vi "RunSimulationBattery-Detector.vi"() -> ()   [LabVIEW 2019]
uses:
  File Exists - Scalar__ogtk.vi
  <vilib>/Utility/file.llb/Read Delimited Spreadsheet (string).vi
  <vilib>/Utility/file.llb/Write Delimited Spreadsheet (string).vi
  <vilib>/Analysis/NI_AALBase.lvlib
panel:
  out "Time to End":cluster{"Time To End":dbl, "unit":string}={"Time To End"=7.502362424242424, "unit"="hr"} {"Time To End" format="%#_4g"}
  in  "A":dbl[](array[numeric])=[0.0, 0.01, 0.01778279410038923, 0.0316227766016838, 0.056234132519034905, 0.1, 0.1778279410038923, 0.31622776601683794, 0.5623413251903492, 1.0, 1.7782794100389228, 3.1622776601683795, 5.623413251903491, 10.0]
  in  "WD":dbl[](array[numeric])=[1.0, 1.5, 2.0, 2.5, 3.0]
  in  "NA":dbl[](array[numeric])=[0.8, 0.85, 0.9, 0.95, 1.0, 1.05, 1.1, 1.15, 1.2000000000000002]
  out "error out":errorcluster
  in  "Target File":path=path "D:/Ian_s Dropbox/Dropbox/PostDoc/Programs/Data/2020-01-15 BigSlab2 Results v01"
  out "Header":string[](array[string])=["Format Version", "Geometry", "Radius (mm)", "Starting Depth (mm)", "G", "Scattering Coefficient", "Absorption Coefficient", "Simulation Grain (mm)", "START Position X", "START Position Y", "START Position Z", "N Photons", "NA", "WD", "LowScatter - N", "LowScatter - Mean Dist", "LowScatter - SD Dist", "LowScatter - I: A = 0.000000", "LowScatter - I: A = 0.010000", "LowScatter - I: A = 0.017783", "LowScatter - I: A = 0.031623", "LowScatter - I: A = 0.056234", "LowScatter - I: A = 0.100000", "LowScatter - I: A = 0.177828", "LowScatter - I: A = 0.316228", "LowScatter - I: A = 0.562341", "LowScatter - I: A = 1.000000", "LowScatter - I: A = 1.778279", "LowScatter - I: A = 3.162278", "LowScatter - I: A = 5.623413", "LowScatter - I: A = 10.000000", "LowScatter - Ave(I): A = 0.000000", "LowScatter - Ave(I): A = 0.010000", "LowScatter - Ave(I): A = 0.017783", "LowScatter - Ave(I): A = 0.031623", "LowScatter - Ave(I): A = 0.056234", "LowScatter - Ave(I): A = 0.100000", "LowScatter - Ave(I): A = 0.177828", "LowScatter - Ave(I): A = 0.316228", "LowScatter - Ave(I): A = 0.562341", "LowScatter - Ave(I): A = 1.000000", "LowScatter - Ave(I): A = 1.778279", "LowScatter - Ave(I): A = 3.162278", "LowScatter - Ave(I): A = 5.623413", "LowScatter - Ave(I): A = 10.000000", "LowScatter - SD(I): A = 0.000000", "LowScatter - SD(I): A = 0.010000", "LowScatter - SD(I): A = 0.017783", "LowScatter - SD(I): A = 0.031623", "LowScatter - SD(I): A = 0.056234", "LowScatter - SD(I): A = 0.100000", "LowScatter - SD(I): A = 0.177828", "LowScatter - SD(I): A = 0.316228", "LowScatter - SD(I): A = 0.562341", "LowScatter - SD(I): A = 1.000000", "LowScatter - SD(I): A = 1.778279", "LowScatter - SD(I): A = 3.162278", "LowScatter - SD(I): A = 5.623413", "LowScatter - SD(I): A = 10.000000"]
  out "transposed array":string[][](array[string])=[["Format Version", "Geometry", "Radius (mm)", "Starting Depth (mm)", "G", "Scattering Coefficient", "Absorption Coefficient", "Simulation Grain (mm)", "START Position X", "START Position Y", "START Position Z"], ["2.0", "SLAB", "5.000000E+0", "1.000000E-9", "9.200000E-1", "0.000000E+0", "1.000000E+0", "1.000000E-4", "0.000000E+0", "0.000000E+0", "5.000000E+0"]]
  out "file names":string[](array[string])=["BigSlab2--SLAB--R5--D0--G0.92--S0--A1--grain0.0001.txt", "BigSlab2--SLAB--R5--D0--G0.92--S0.1--A1--grain0.0001.txt", "BigSlab2--SLAB--R5--D0--G0.92--S0.177828--A1--grain0.0001.txt", "BigSlab2--SLAB--R5--D0--G0.92--S0.316228--A1--grain0.0001.txt", "BigSlab2--SLAB--R5--D0--G0.92--S0.562341--A1--grain0.0001.txt", "BigSlab2--SLAB--R5--D0--G0.92--S1--A1--grain0.0001.txt", "BigSlab2--SLAB--R5--D0--G0.92--S1.778279--A1--grain0.0001.txt", "BigSlab2--SLAB--R5--D0--G0.92--S10--A1--grain0.0001.txt", "BigSlab2--SLAB--R5--D0--G0.92--S3.162278--A1--grain0.0001.txt", "BigSlab2--SLAB--R5--D0--G0.92--S5.623413--A1--grain0.0001.txt", "BigSlab2--SLAB--R5--D0.1--G0.92--S0--A1--grain0.0001.txt", "BigSlab2--SLAB--R5--D0.1--G0.92--S0.1--A1--grain0.0001.txt", "BigSlab2--SLAB--R5--D0.1--G0.92--S0.177828--A1--grain0.0001.txt", "BigSlab2--SLAB--R5--D0.1--G0.92--S0.316228--A1--grain0.0001.txt", "BigSlab2--SLAB--R5--D0.1--G0.92--S0.562341--A1--grain0.0001.txt", "BigSlab2--SLAB--R5--D0.1--G0.92--S1--A1--grain0.0001.txt", "BigSlab2--SLAB--R5--D0.1--G0.92--S1.778279--A1--grain0.0001.txt", "BigSlab2--SLAB--R5--D0.1--G0.92--S10--A1--grain0.0001.txt", "BigSlab2--SLAB--R5--D0.1--G0.92--S3.162278--A1--grain0.0001.txt", "BigSlab2--SLAB--R5--D0.1--G0.92--S5.623413--A1--grain0.0001.txt", "BigSlab2--SLAB--R5--D0.2--G0.92--S0--A1--grain0.0001.txt", "BigSlab2--SLAB--R5--D0.2--G0.92--S0.1--A1--grain0.0001.txt", "BigSlab2--SLAB--R5--D0.2--G0.92--S0.177828--A1--grain0.0001.txt", "BigSlab2--SLAB--R5--D0.2--G0.92--S0.316228--A1--grain0.0001.txt", "BigSlab2--SLAB--R5--D0.2--G0.92--S0.562341--A1--grain0.0001.txt", "BigSlab2--SLAB--R5--D0.2--G0.92--S1--A1--grain0.0001.txt", "BigSlab2--SLAB--R5--D0.2--G0.92--S1.778279--A1--grain0.0001.txt", "BigSlab2--SLAB--R5--D0.2--G0.92--S10--A1--grain0.0001.txt", "BigSlab2--SLAB--R5--D0.2--G0.92--S3.162278--A1--grain0.0001.txt", "BigSlab2--SLAB--R5--D0.2--G0.92--S5.623413--A1--grain0.0001.txt", "BigSlab2--SLAB--R5--D0.3--G0.92--S0--A1--grain0.0001.txt", "BigSlab2--SLAB--R5--D0.3--G0.92--S0.1--A1--grain0.0001.txt", "BigSlab2--SLAB--R5--D0.3--G0.92--S0.177828--A1--grain0.0001.txt", "BigSlab2--SLAB--R5--D0.3--G0.92--S0.316228--A1--grain0.0001.txt", "BigSlab2--SLAB--R5--D0.3--G0.92--S0.562341--A1--grain0.0001.txt", "BigSlab2--SLAB--R5--D0.3--G0.92--S1--A1--grain0.0001.txt", "BigSlab2--SLAB--R5--D0.3--G0.92--S1.778279--A1--grain0.0001.txt", "BigSlab2--SLAB--R5--D0.3--G0.92--S10--A1--grain0.0001.txt", "BigSlab2--SLAB--R5--D0.3--G0.92--S3.162278--A1--grain0.0001.txt", "BigSlab2--SLAB--R5--D0.3--G0.92--S5.623413--A1--grain0.0001.txt", "BigSlab2--SLAB--R5--D0.4--G0.92--S0--A1--grain0.0001.txt", "BigSlab2--SLAB--R5--D0.4--G0.92--S0.1--A1--grain0.0001.txt", "BigSlab2--SLAB--R5--D0.4--G0.92--S0.177828--A1--grain0.0001.txt", "BigSlab2--SLAB--R5--D0.4--G0.92--S0.316228--A1--grain0.0001.txt", "BigSlab2--SLAB--R5--D0.4--G0.92--S0.562341--A1--grain0.0001.txt", "BigSlab2--SLAB--R5--D0.4--G0.92--S1--A1--grain0.0001.txt", "BigSlab2--SLAB--R5--D0.4--G0.92--S1.778279--A1--grain0.0001.txt", "BigSlab2--SLAB--R5--D0.4--G0.92--S10--A1--grain0.0001.txt", "BigSlab2--SLAB--R5--D0.4--G0.92--S3.162278--A1--grain0.0001.txt", "BigSlab2--SLAB--R5--D0.4--G0.92--S5.623413--A1--grain0.0001.txt", "BigSlab2--SLAB--R5--D0.5--G0.92--S0--A1--grain0.0001.txt", "BigSlab2--SLAB--R5--D0.5--G0.92--S0.1--A1--grain0.0001.txt", "BigSlab2--SLAB--R5--D0.5--G0.92--S0.177828--A1--grain0.0001.txt", "BigSlab2--SLAB--R5--D0.5--G0.92--S0.316228--A1--grain0.0001.txt", "BigSlab2--SLAB--R5--D0.5--G0.92--S0.562341--A1--grain0.0001.txt", "BigSlab2--SLAB--R5--D0.5--G0.92--S1--A1--grain0.0001.txt", "BigSlab2--SLAB--R5--D0.5--G0.92--S1.778279--A1--grain0.0001.txt", "BigSlab2--SLAB--R5--D0.5--G0.92--S10--A1--grain0.0001.txt", "BigSlab2--SLAB--R5--D0.5--G0.92--S3.162278--A1--grain0.0001.txt", "BigSlab2--SLAB--R5--D0.5--G0.92--S5.623413--A1--grain0.0001.txt", "BigSlab2--SLAB--R5--D0.6--G0.92--S0--A1--grain0.0001.txt", "BigSlab2--SLAB--R5--D0.6--G0.92--S0.1--A1--grain0.0001.txt", "BigSlab2--SLAB--R5--D0.6--G0.92--S0.177828--A1--grain0.0001.txt", "BigSlab2--SLAB--R5--D0.6--G0.92--S0.316228--A1--grain0.0001.txt", "BigSlab2--SLAB--R5--D0.6--G0.92--S0.562341--A1--grain0.0001.txt", "BigSlab2--SLAB--R5--D0.6--G0.92--S1--A1--grain0.0001.txt", "BigSlab2--SLAB--R5--D0.6--G0.92--S1.778279--A1--grain0.0001.txt", "BigSlab2--SLAB--R5--D0.6--G0.92--S10--A1--grain0.0001.txt", "BigSlab2--SLAB--R5--D0.6--G0.92--S3.162278--A1--grain0.0001.txt", "BigSlab2--SLAB--R5--D0.6--G0.92--S5.623413--A1--grain0.0001.txt", "BigSlab2--SLAB--R5--D0.7--G0.92--S0--A1--grain0.0001.txt", "BigSlab2--SLAB--R5--D0.7--G0.92--S0.1--A1--grain0.0001.txt", "BigSlab2--SLAB--R5--D0.7--G0.92--S0.177828--A1--grain0.0001.txt", "BigSlab2--SLAB--R5--D0.7--G0.92--S0.316228--A1--grain0.0001.txt", "BigSlab2--SLAB--R5--D0.7--G0.92--S0.562341--A1--grain0.0001.txt", "BigSlab2--SLAB--R5--D0.7--G0.92--S1--A1--grain0.0001.txt", "BigSlab2--SLAB--R5--D0.7--G0.92--S1.778279--A1--grain0.0001.txt", "BigSlab2--SLAB--R5--D0.7--G0.92--S10--A1--grain0.0001.txt", "BigSlab2--SLAB--R5--D0.7--G0.92--S3.162278--A1--grain0.0001.txt", "BigSlab2--SLAB--R5--D0.7--G0.92--S5.623413--A1--grain0.0001.txt", "BigSlab2--SLAB--R5--D0.8--G0.92--S0--A1--grain0.0001.txt", "BigSlab2--SLAB--R5--D0.8--G0.92--S0.1--A1--grain0.0001.txt", "BigSlab2--SLAB--R5--D0.8--G0.92--S0.177828--A1--grain0.0001.txt", "BigSlab2--SLAB--R5--D0.8--G0.92--S0.316228--A1--grain0.0001.txt", "BigSlab2--SLAB--R5--D0.8--G0.92--S0.562341--A1--grain0.0001.txt", "BigSlab2--SLAB--R5--D0.8--G0.92--S1--A1--grain0.0001.txt", "BigSlab2--SLAB--R5--D0.8--G0.92--S1.778279--A1--grain0.0001.txt", "BigSlab2--SLAB--R5--D0.8--G0.92--S10--A1--grain0.0001.txt", "BigSlab2--SLAB--R5--D0.8--G0.92--S3.162278--A1--grain0.0001.txt", "BigSlab2--SLAB--R5--D0.8--G0.92--S5.623413--A1--grain0.0001.txt", "BigSlab2--SLAB--R5--D0.9--G0.92--S0--A1--grain0.0001.txt", "BigSlab2--SLAB--R5--D0.9--G0.92--S0.1--A1--grain0.0001.txt", "BigSlab2--SLAB--R5--D0.9--G0.92--S0.177828--A1--grain0.0001.txt", "BigSlab2--SLAB--R5--D0.9--G0.92--S0.316228--A1--grain0.0001.txt", "BigSlab2--SLAB--R5--D0.9--G0.92--S0.562341--A1--grain0.0001.txt", "BigSlab2--SLAB--R5--D0.9--G0.92--S1--A1--grain0.0001.txt", "BigSlab2--SLAB--R5--D0.9--G0.92--S1.778279--A1--grain0.0001.txt", "BigSlab2--SLAB--R5--D0.9--G0.92--S10--A1--grain0.0001.txt", "BigSlab2--SLAB--R5--D0.9--G0.92--S3.162278--A1--grain0.0001.txt", "BigSlab2--SLAB--R5--D0.9--G0.92--S5.623413--A1--grain0.0001.txt", "BigSlab2--SLAB--R5--D1--G0.92--S0--A1--grain0.0001.txt", "BigSlab2--SLAB--R5--D1--G0.92--S0.1--A1--grain0.0001.txt", "BigSlab2--SLAB--R5--D1--G0.92--S0.177828--A1--grain0.0001.txt", "BigSlab2--SLAB--R5--D1--G0.92--S0.316228--A1--grain0.0001.txt", "BigSlab2--SLAB--R5--D1--G0.92--S0.562341--A1--grain0.0001.txt", "BigSlab2--SLAB--R5--D1--G0.92--S1--A1--grain0.0001.txt", "BigSlab2--SLAB--R5--D1--G0.92--S1.778279--A1--grain0.0001.txt", "BigSlab2--SLAB--R5--D1--G0.92--S10--A1--grain0.0001.txt", "BigSlab2--SLAB--R5--D1--G0.92--S3.162278--A1--grain0.0001.txt", "BigSlab2--SLAB--R5--D1--G0.92--S5.623413--A1--grain0.0001.txt", "BigSlab2--SLAB--R5--D1.1--G0.92--S0--A1--grain0.0001.txt", "BigSlab2--SLAB--R5--D1.1--G0.92--S0.1--A1--grain0.0001.txt", "BigSlab2--SLAB--R5--D1.1--G0.92--S0.177828--A1--grain0.0001.txt", "BigSlab2--SLAB--R5--D1.1--G0.92--S0.316228--A1--grain0.0001.txt", "BigSlab2--SLAB--R5--D1.1--G0.92--S0.562341--A1--grain0.0001.txt", "BigSlab2--SLAB--R5--D1.1--G0.92--S1--A1--grain0.0001.txt", "BigSlab2--SLAB--R5--D1.1--G0.92--S1.778279--A1--grain0.0001.txt", "BigSlab2--SLAB--R5--D1.1--G0.92--S10--A1--grain0.0001.txt", "BigSlab2--SLAB--R5--D1.1--G0.92--S3.162278--A1--grain0.0001.txt", "BigSlab2--SLAB--R5--D1.1--G0.92--S5.623413--A1--grain0.0001.txt", "BigSlab2--SLAB--R5--D1.2--G0.92--S0--A1--grain0.0001.txt", "BigSlab2--SLAB--R5--D1.2--G0.92--S0.1--A1--grain0.0001.txt", "BigSlab2--SLAB--R5--D1.2--G0.92--S0.177828--A1--grain0.0001.txt", "BigSlab2--SLAB--R5--D1.2--G0.92--S0.316228--A1--grain0.0001.txt", "BigSlab2--SLAB--R5--D1.2--G0.92--S0.562341--A1--grain0.0001.txt", "BigSlab2--SLAB--R5--D1.2--G0.92--S1--A1--grain0.0001.txt", "BigSlab2--SLAB--R5--D1.2--G0.92--S1.778279--A1--grain0.0001.txt", "BigSlab2--SLAB--R5--D1.2--G0.92--S10--A1--grain0.0001.txt", "BigSlab2--SLAB--R5--D1.2--G0.92--S3.162278--A1--grain0.0001.txt", "BigSlab2--SLAB--R5--D1.2--G0.92--S5.623413--A1--grain0.0001.txt", "BigSlab2--SLAB--R5--D1.3--G0.92--S0--A1--grain0.0001.txt", "BigSlab2--SLAB--R5--D1.3--G0.92--S0.1--A1--grain0.0001.txt", "BigSlab2--SLAB--R5--D1.3--G0.92--S0.177828--A1--grain0.0001.txt", "BigSlab2--SLAB--R5--D1.3--G0.92--S0.316228--A1--grain0.0001.txt", "BigSlab2--SLAB--R5--D1.3--G0.92--S0.562341--A1--grain0.0001.txt", "BigSlab2--SLAB--R5--D1.3--G0.92--S1--A1--grain0.0001.txt", "BigSlab2--SLAB--R5--D1.3--G0.92--S1.778279--A1--grain0.0001.txt", "BigSlab2--SLAB--R5--D1.3--G0.92--S10--A1--grain0.0001.txt", "BigSlab2--SLAB--R5--D1.3--G0.92--S3.162278--A1--grain0.0001.txt", "BigSlab2--SLAB--R5--D1.3--G0.92--S5.623413--A1--grain0.0001.txt", "BigSlab2--SLAB--R5--D1.4--G0.92--S0--A1--grain0.0001.txt", "BigSlab2--SLAB--R5--D1.4--G0.92--S0.1--A1--grain0.0001.txt", "BigSlab2--SLAB--R5--D1.4--G0.92--S0.177828--A1--grain0.0001.txt", "BigSlab2--SLAB--R5--D1.4--G0.92--S0.316228--A1--grain0.0001.txt", "BigSlab2--SLAB--R5--D1.4--G0.92--S0.562341--A1--grain0.0001.txt", "BigSlab2--SLAB--R5--D1.4--G0.92--S1--A1--grain0.0001.txt", "BigSlab2--SLAB--R5--D1.4--G0.92--S1.778279--A1--grain0.0001.txt", "BigSlab2--SLAB--R5--D1.4--G0.92--S10--A1--grain0.0001.txt", "BigSlab2--SLAB--R5--D1.4--G0.92--S3.162278--A1--grain0.0001.txt", "BigSlab2--SLAB--R5--D1.4--G0.92--S5.623413--A1--grain0.0001.txt", "BigSlab2--SLAB--R5--D1.5--G0.92--S0--A1--grain0.0001.txt", "BigSlab2--SLAB--R5--D1.5--G0.92--S0.1--A1--grain0.0001.txt", "BigSlab2--SLAB--R5--D1.5--G0.92--S0.177828--A1--grain0.0001.txt", "BigSlab2--SLAB--R5--D1.5--G0.92--S0.316228--A1--grain0.0001.txt", "BigSlab2--SLAB--R5--D1.5--G0.92--S0.562341--A1--grain0.0001.txt", "BigSlab2--SLAB--R5--D1.5--G0.92--S1--A1--grain0.0001.txt", "BigSlab2--SLAB--R5--D1.5--G0.92--S1.778279--A1--grain0.0001.txt", "BigSlab2--SLAB--R5--D1.5--G0.92--S10--A1--grain0.0001.txt", "BigSlab2--SLAB--R5--D1.5--G0.92--S3.162278--A1--grain0.0001.txt", "BigSlab2--SLAB--R5--D1.5--G0.92--S5.623413--A1--grain0.0001.txt", "BigSlab2--SLAB--R5--D1.6--G0.92--S0--A1--grain0.0001.txt", "BigSlab2--SLAB--R5--D1.6--G0.92--S0.1--A1--grain0.0001.txt", "BigSlab2--SLAB--R5--D1.6--G0.92--S0.177828--A1--grain0.0001.txt", "BigSlab2--SLAB--R5--D1.6--G0.92--S0.316228--A1--grain0.0001.txt", "BigSlab2--SLAB--R5--D1.6--G0.92--S0.562341--A1--grain0.0001.txt", "BigSlab2--SLAB--R5--D1.6--G0.92--S1--A1--grain0.0001.txt", "BigSlab2--SLAB--R5--D1.6--G0.92--S1.778279--A1--grain0.0001.txt", "BigSlab2--SLAB--R5--D1.6--G0.92--S10--A1--grain0.0001.txt", "BigSlab2--SLAB--R5--D1.6--G0.92--S3.162278--A1--grain0.0001.txt", "BigSlab2--SLAB--R5--D1.6--G0.92--S5.623413--A1--grain0.0001.txt", "BigSlab2--SLAB--R5--D1.7--G0.92--S0--A1--grain0.0001.txt", "BigSlab2--SLAB--R5--D1.7--G0.92--S0.1--A1--grain0.0001.txt", "BigSlab2--SLAB--R5--D1.7--G0.92--S0.177828--A1--grain0.0001.txt", "BigSlab2--SLAB--R5--D1.7--G0.92--S0.316228--A1--grain0.0001.txt", "BigSlab2--SLAB--R5--D1.7--G0.92--S0.562341--A1--grain0.0001.txt", "BigSlab2--SLAB--R5--D1.7--G0.92--S1--A1--grain0.0001.txt", "BigSlab2--SLAB--R5--D1.7--G0.92--S1.778279--A1--grain0.0001.txt", "BigSlab2--SLAB--R5--D1.7--G0.92--S10--A1--grain0.0001.txt", "BigSlab2--SLAB--R5--D1.7--G0.92--S3.162278--A1--grain0.0001.txt", "BigSlab2--SLAB--R5--D1.7--G0.92--S5.623413--A1--grain0.0001.txt", "BigSlab2--SLAB--R5--D1.8--G0.92--S0--A1--grain0.0001.txt", "BigSlab2--SLAB--R5--D1.8--G0.92--S0.1--A1--grain0.0001.txt", "BigSlab2--SLAB--R5--D1.8--G0.92--S0.177828--A1--grain0.0001.txt", "BigSlab2--SLAB--R5--D1.8--G0.92--S0.316228--A1--grain0.0001.txt", "BigSlab2--SLAB--R5--D1.8--G0.92--S0.562341--A1--grain0.0001.txt", "BigSlab2--SLAB--R5--D1.8--G0.92--S1--A1--grain0.0001.txt", "BigSlab2--SLAB--R5--D1.8--G0.92--S1.778279--A1--grain0.0001.txt", "BigSlab2--SLAB--R5--D1.8--G0.92--S10--A1--grain0.0001.txt", "BigSlab2--SLAB--R5--D1.8--G0.92--S3.162278--A1--grain0.0001.txt", "BigSlab2--SLAB--R5--D1.8--G0.92--S5.623413--A1--grain0.0001.txt", "BigSlab2--SLAB--R5--D1.9--G0.92--S0--A1--grain0.0001.txt", "BigSlab2--SLAB--R5--D1.9--G0.92--S0.1--A1--grain0.0001.txt", "BigSlab2--SLAB--R5--D1.9--G0.92--S0.177828--A1--grain0.0001.txt", "BigSlab2--SLAB--R5--D1.9--G0.92--S0.316228--A1--grain0.0001.txt", "BigSlab2--SLAB--R5--D1.9--G0.92--S0.562341--A1--grain0.0001.txt", "BigSlab2--SLAB--R5--D1.9--G0.92--S1--A1--grain0.0001.txt", "BigSlab2--SLAB--R5--D1.9--G0.92--S1.778279--A1--grain0.0001.txt", "BigSlab2--SLAB--R5--D1.9--G0.92--S10--A1--grain0.0001.txt", "BigSlab2--SLAB--R5--D1.9--G0.92--S3.162278--A1--grain0.0001.txt", "BigSlab2--SLAB--R5--D1.9--G0.92--S5.623413--A1--grain0.0001.txt", "BigSlab2--SLAB--R5--D2--G0.92--S0--A1--grain0.0001.txt", "BigSlab2--SLAB--R5--D2--G0.92--S0.1--A1--grain0.0001.txt", "BigSlab2--SLAB--R5--D2--G0.92--S0.177828--A1--grain0.0001.txt", "BigSlab2--SLAB--R5--D2--G0.92--S0.316228--A1--grain0.0001.txt", "BigSlab2--SLAB--R5--D2--G0.92--S0.562341--A1--grain0.0001.txt", "BigSlab2--SLAB--R5--D2--G0.92--S1--A1--grain0.0001.txt", "BigSlab2--SLAB--R5--D2--G0.92--S1.778279--A1--grain0.0001.txt", "BigSlab2--SLAB--R5--D2--G0.92--S10--A1--grain0.0001.txt", "BigSlab2--SLAB--R5--D2--G0.92--S3.162278--A1--grain0.0001.txt", "BigSlab2--SLAB--R5--D2--G0.92--S5.623413--A1--grain0.0001.txt", "BigSlab2--SLAB--R5--D2.5--G0.92--S0--A1--grain0.0001.txt", "BigSlab2--SLAB--R5--D2.5--G0.92--S0.1--A1--grain0.0001.txt", "BigSlab2--SLAB--R5--D2.5--G0.92--S0.177828--A1--grain0.0001.txt", "BigSlab2--SLAB--R5--D2.5--G0.92--S0.316228--A1--grain0.0001.txt", "BigSlab2--SLAB--R5--D2.5--G0.92--S0.562341--A1--grain0.0001.txt", "BigSlab2--SLAB--R5--D2.5--G0.92--S1--A1--grain0.0001.txt", "BigSlab2--SLAB--R5--D2.5--G0.92--S1.778279--A1--grain0.0001.txt", "BigSlab2--SLAB--R5--D2.5--G0.92--S10--A1--grain0.0001.txt", "BigSlab2--SLAB--R5--D2.5--G0.92--S3.162278--A1--grain0.0001.txt", "BigSlab2--SLAB--R5--D2.5--G0.92--S5.623413--A1--grain0.0001.txt", "BigSlab2--SLAB--R5--D3--G0.92--S0--A1--grain0.0001.txt", "BigSlab2--SLAB--R5--D3--G0.92--S0.1--A1--grain0.0001.txt", "BigSlab2--SLAB--R5--D3--G0.92--S0.177828--A1--grain0.0001.txt", "BigSlab2--SLAB--R5--D3--G0.92--S0.316228--A1--grain0.0001.txt", "BigSlab2--SLAB--R5--D3--G0.92--S0.562341--A1--grain0.0001.txt", "BigSlab2--SLAB--R5--D3--G0.92--S1--A1--grain0.0001.txt", "BigSlab2--SLAB--R5--D3--G0.92--S1.778279--A1--grain0.0001.txt", "BigSlab2--SLAB--R5--D3--G0.92--S10--A1--grain0.0001.txt", "BigSlab2--SLAB--R5--D3--G0.92--S3.162278--A1--grain0.0001.txt", "BigSlab2--SLAB--R5--D3--G0.92--S5.623413--A1--grain0.0001.txt", "BigSlab2--SLAB--R5--D3.5--G0.92--S0--A1--grain0.0001.txt", "BigSlab2--SLAB--R5--D3.5--G0.92--S0.1--A1--grain0.0001.txt", "BigSlab2--SLAB--R5--D3.5--G0.92--S0.177828--A1--grain0.0001.txt", "BigSlab2--SLAB--R5--D3.5--G0.92--S0.316228--A1--grain0.0001.txt", "BigSlab2--SLAB--R5--D3.5--G0.92--S0.562341--A1--grain0.0001.txt", "BigSlab2--SLAB--R5--D3.5--G0.92--S1--A1--grain0.0001.txt", "BigSlab2--SLAB--R5--D3.5--G0.92--S1.778279--A1--grain0.0001.txt", "BigSlab2--SLAB--R5--D3.5--G0.92--S10--A1--grain0.0001.txt", "BigSlab2--SLAB--R5--D3.5--G0.92--S3.162278--A1--grain0.0001.txt", "BigSlab2--SLAB--R5--D3.5--G0.92--S5.623413--A1--grain0.0001.txt", "BigSlab2--SLAB--R5--D4--G0.92--S0--A1--grain0.0001.txt", "BigSlab2--SLAB--R5--D4--G0.92--S0.1--A1--grain0.0001.txt", "BigSlab2--SLAB--R5--D4--G0.92--S0.177828--A1--grain0.0001.txt", "BigSlab2--SLAB--R5--D4--G0.92--S0.316228--A1--grain0.0001.txt", "BigSlab2--SLAB--R5--D4--G0.92--S0.562341--A1--grain0.0001.txt", "BigSlab2--SLAB--R5--D4--G0.92--S1--A1--grain0.0001.txt", "BigSlab2--SLAB--R5--D4--G0.92--S1.778279--A1--grain0.0001.txt", "BigSlab2--SLAB--R5--D4--G0.92--S10--A1--grain0.0001.txt", "BigSlab2--SLAB--R5--D4--G0.92--S3.162278--A1--grain0.0001.txt", "BigSlab2--SLAB--R5--D4--G0.92--S5.623413--A1--grain0.0001.txt", "BigSlab2--SLAB--R5--D4.5--G0.92--S0--A1--grain0.0001.txt", "BigSlab2--SLAB--R5--D4.5--G0.92--S0.1--A1--grain0.0001.txt", "BigSlab2--SLAB--R5--D4.5--G0.92--S0.177828--A1--grain0.0001.txt", "BigSlab2--SLAB--R5--D4.5--G0.92--S0.316228--A1--grain0.0001.txt", "BigSlab2--SLAB--R5--D4.5--G0.92--S0.562341--A1--grain0.0001.txt", "BigSlab2--SLAB--R5--D4.5--G0.92--S1--A1--grain0.0001.txt", "BigSlab2--SLAB--R5--D4.5--G0.92--S1.778279--A1--grain0.0001.txt", "BigSlab2--SLAB--R5--D4.5--G0.92--S10--A1--grain0.0001.txt", "BigSlab2--SLAB--R5--D4.5--G0.92--S3.162278--A1--grain0.0001.txt", "BigSlab2--SLAB--R5--D4.5--G0.92--S5.623413--A1--grain0.0001.txt", "BigSlab2--SLAB--R5--D5--G0.92--S0--A1--grain0.0001.txt", "BigSlab2--SLAB--R5--D5--G0.92--S0.1--A1--grain0.0001.txt", "BigSlab2--SLAB--R5--D5--G0.92--S0.177828--A1--grain0.0001.txt", "BigSlab2--SLAB--R5--D5--G0.92--S0.316228--A1--grain0.0001.txt", "BigSlab2--SLAB--R5--D5--G0.92--S0.562341--A1--grain0.0001.txt", "BigSlab2--SLAB--R5--D5--G0.92--S1--A1--grain0.0001.txt", "BigSlab2--SLAB--R5--D5--G0.92--S1.778279--A1--grain0.0001.txt", "BigSlab2--SLAB--R5--D5--G0.92--S10--A1--grain0.0001.txt", "BigSlab2--SLAB--R5--D5--G0.92--S3.162278--A1--grain0.0001.txt", "BigSlab2--SLAB--R5--D5--G0.92--S5.623413--A1--grain0.0001.txt"]
  out "Percent Complete":dbl(slide)=0.0018106995884773663 scale=0.0..1.0
  in  "Folder of Media Simulations":path=path "D:/Ian_s Dropbox/Dropbox/PostDoc/Programs/Data/2020-01-15 BigSlab2"
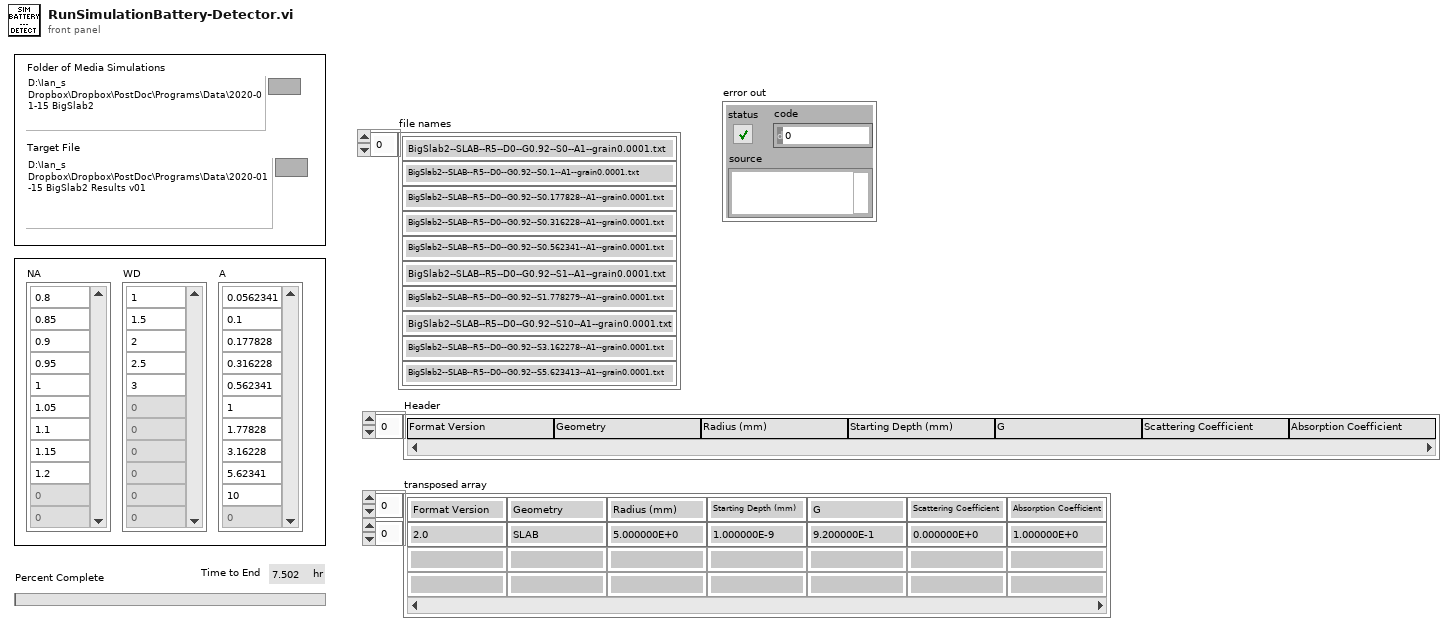
[diagram p1: front panel]
types:
  T1 = enum16{"Delete Empty Rows", "Delete Empty Columns"}
  T2 = typedef "PhotonState--Enum.ctl" = enum16{"Detected - Low Scattering", "Detected - High Scattering", "Undetected"}
  T3 = cluster{"Photon State":T2, "Phi":dbl, "String":dbl}
  T4 = cluster{"Photon State":T2, "Phi":dbl, "String":dbl}[]
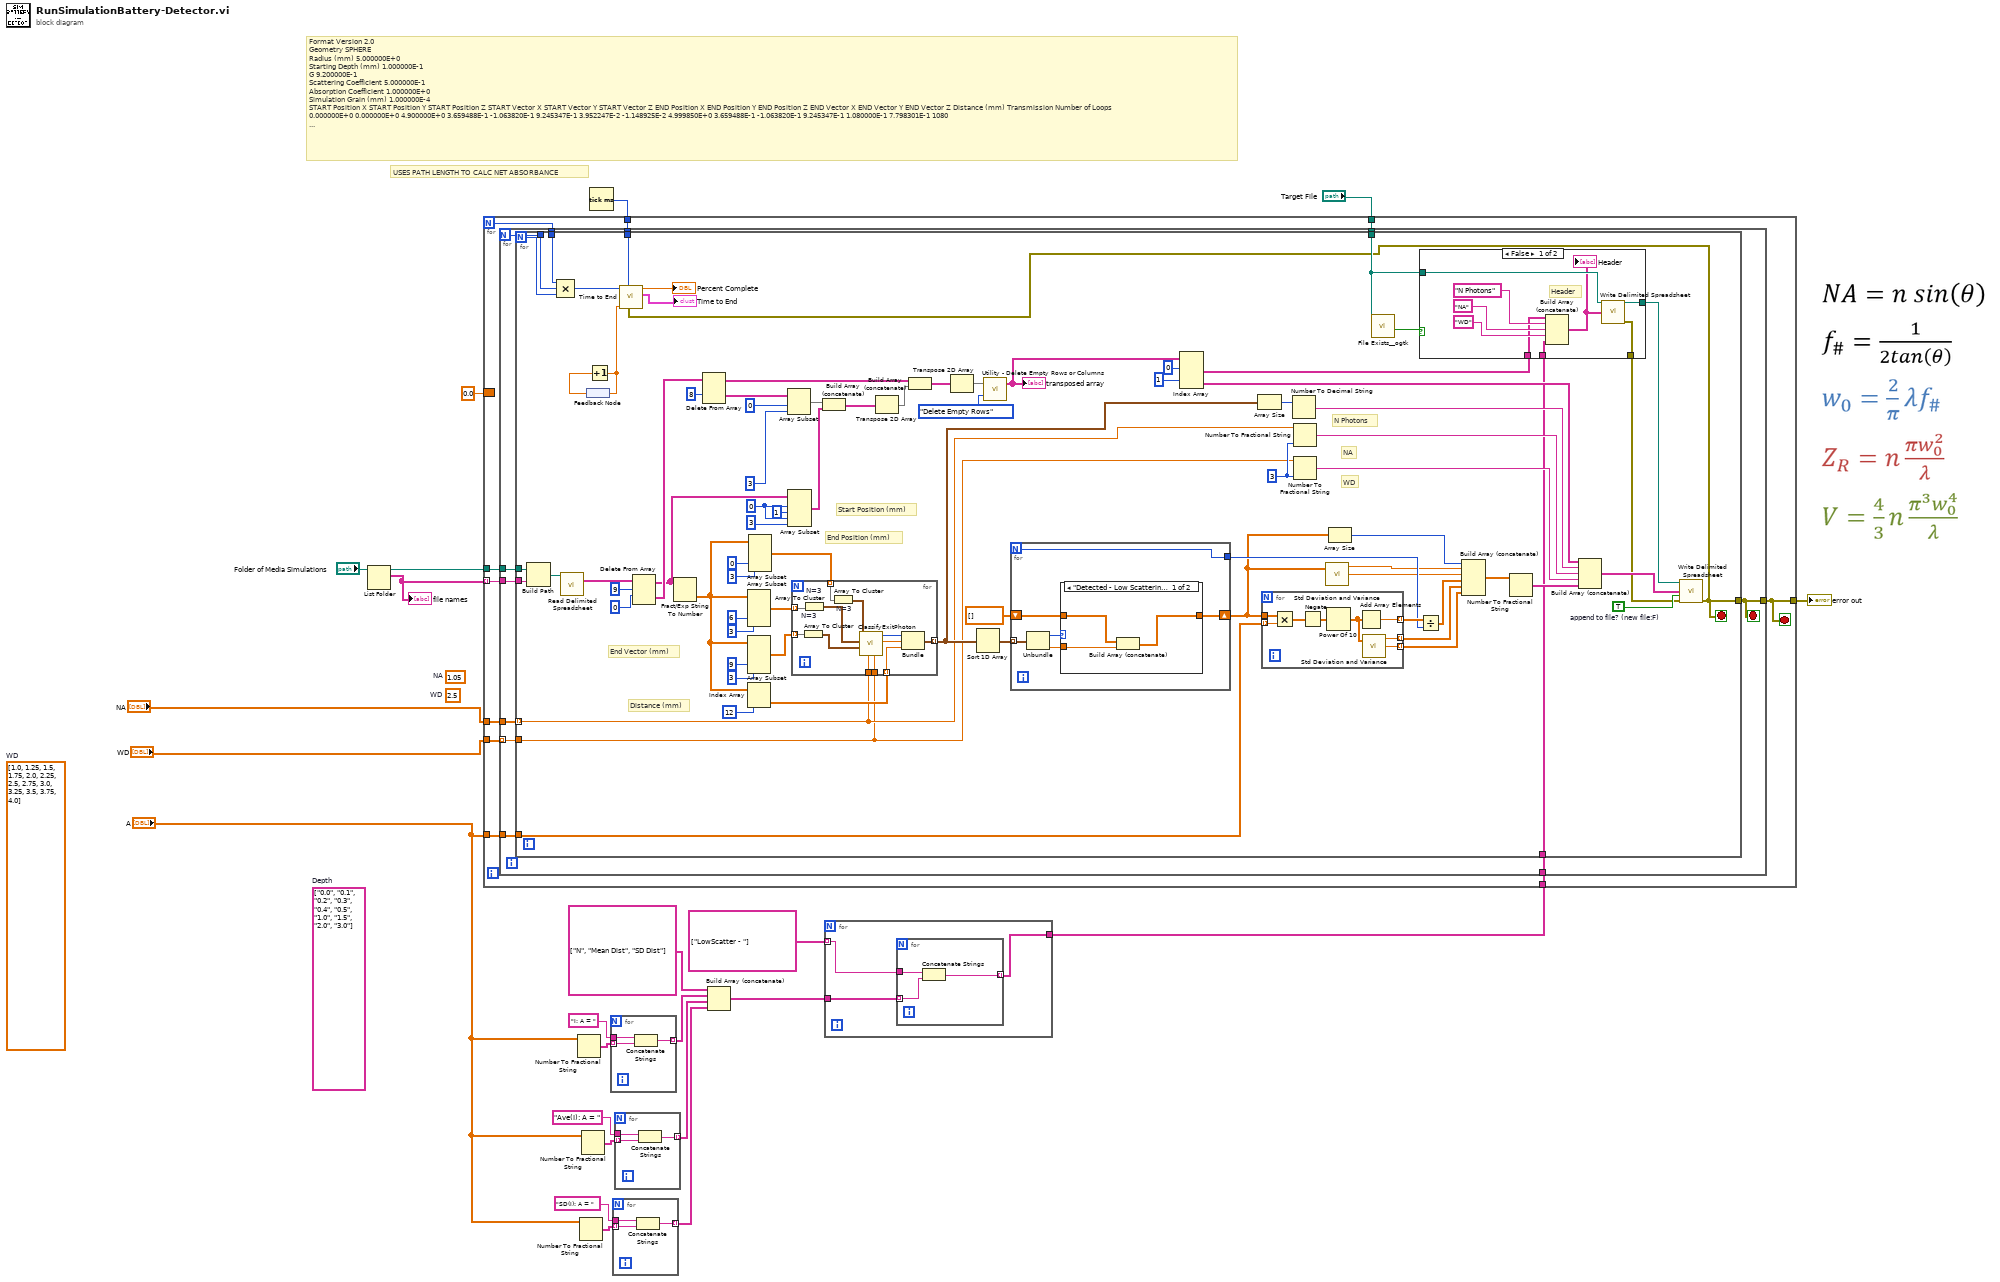
[diagram p0: block diagram]
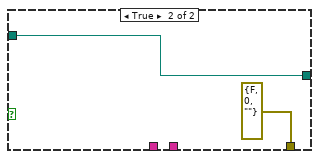
[diagram p2: hidden frame]
diagram:
  (unwired) dbl[] [1.0, 1.25, 1.5, 1.75, 2.0, 2.25, 2.5, 2.75, 3.0, 3.25, 3.5, 3.75, 4.0]  # WD
  (unwired) 2.5  # WD
  (unwired) 1.05  # NA
  (unwired) string[] ["0.0", "0.1", "0.2", "0.3", "0.4", "0.5", "1.0", "1.5", "2.0", "3.0"]  # Depth
  # "Format Version\t2.0\t\t\t\t\t\t\t\t\t\t\t\t\t\nGeometry\tSPHERE\t\t\t\t\t\t\t\t\t\t\t\t\t\nRadius (mm)\t5.000000E+0\t\t\t\t\t\t\t\t\t\t\t\t\t\nStarting Depth (mm)\t1.000000E-1\t\t\t\t\t\t\t\t\t\t\t\t\t\nG\t9.200000E-1\t\t\t\t\t\t\t\t\t\t\t\t\t\nScattering Coefficient\t5.000000E-1\t\t\t\t\t\t\t\t\t\t\t\t\t\nAbsorption Coefficient\t1.000000E+0\t\t\t\t\t\t\t\t\t\t\t\t\t\nSimulation Grain (mm)\t1.000000E-4\t\t\t\t\t\t\t\t\t\t\t\t\t\nSTART Position X\tSTART Position Y\tSTART Position Z\tSTART Vector X\tSTART Vector Y\tSTART Vector Z\tEND Position X\tEND Position Y\tEND Position Z\tEND Vector X\tEND Vector Y\tEND Vector Z\tDistance (mm)\tTransmission\tNumber of Loops\n0.000000E+0\t0.000000E+0\t4.900000E+0\t3.659488E-1\t-1.063820E-1\t9.245347E-1\t3.952247E-2\t-1.148925E-2\t4.999850E+0\t3.659488E-1\t-1.063820E-1\t9.245347E-1\t1.080000E-1\t7.798301E-1\t1080\n..."
  # "USES PATH LENGTH TO CALC NET ABSORBANCE"
  n1 = List Folder(path="Folder of Media Simulations") -> (path out=w21:path, filenames=w22:string[])  [unwired: 3 in, 2 out]
  "file names" <- w22
  n2 = Number To Fractional String(number="A") -> (F-format string=w20:string[])  [unwired: 3 in]
  n3 = Number To Fractional String(number="A") -> (F-format string=w12:string[])  [unwired: 3 in]
  n4 = Number To Fractional String(number="A") -> (F-format string=w13:string[])  [unwired: 3 in]
  n5 = Tick Count (ms)() -> (millisecond timer value=w1:u32)
  n6 = for {
    tunnel: w20 -> [w26] mode=indexing
    tunnel: "I: A = " ("string") -> [w25]
    tunnel: [w24] -> w17 mode=indexing
    n7 = Concatenate Strings(w25, w26) -> (w24:string)
  }
  n8 = for {
    tunnel: w12 -> [w29] mode=indexing
    tunnel: "SD(I): A = " ("string") -> [w28]
    tunnel: [w27] -> w9 mode=indexing
    n9 = Concatenate Strings(w28, w29) -> (w27:string)
  }
  n10 = for {
    tunnel: w13 -> [w32] mode=indexing
    tunnel: "Ave(I): A = " ("string") -> [w31]
    tunnel: [w30] -> w10 mode=indexing
    n11 = Concatenate Strings(w31, w32) -> (w30:string)
  }
  n12 = Build Array (concatenate)(string[] ["N", "Mean Dist", "SD Dist"] ("Array 2"), w17, w10, w9) -> (w15:string[])
  n13 = for {
    tunnel: string[] ["LowScatter - "] ("Array 2") -> [w35] mode=indexing
    tunnel: w15 -> [w34]
    tunnel: [w33] -> w4
    n14 = for {
      tunnel: w35 -> [w38]
      tunnel: w34 -> [w37] mode=indexing
      tunnel: [w36] -> w33 mode=indexing
      n15 = Concatenate Strings(w38, w37) -> (w36:string)
    }
  }
  n16 = for {
    N -> [w43]
    tunnel: w21 -> [w48]
    tunnel: "NA" -> [w47]
    tunnel: "A" -> [w44]
    tunnel: w22 -> [w46] mode=indexing
    tunnel: "WD" -> [w45]
    border: 0.0 -> [_]
    tunnel: [w42] -> w3
    tunnel: "Target File" -> [w41]
    tunnel: w4 -> [w40]
    tunnel: w1 -> [w39]
    stop <- w42 stop-if-true
    n17 = for {
      N -> [w54]
      tunnel: w48 -> [w59]
      tunnel: w47 -> [w58]
      tunnel: w46 -> [w57]
      tunnel: w45 -> [w56] mode=indexing
      tunnel: w44 -> [w55]
      tunnel: w43 -> [w53]
      tunnel: [w52] -> w42
      tunnel: w41 -> [w51]
      tunnel: w40 -> [w50]
      tunnel: w39 -> [w49]
      stop <- w52 stop-if-true
      n18 = for {
        N -> [w86]
        tunnel: w59 -> [w138]
        tunnel: w58 -> [w89] mode=indexing
        tunnel: w57 -> [w126]
        tunnel: w56 -> [w88]
        tunnel: w55 -> [w103]
        tunnel: w54 -> [w85]
        tunnel: w53 -> [w84]
        tunnel: [w64] -> w52
        tunnel: w51 -> [w70]
        tunnel: w50 -> [w72]
        tunnel: w49 -> [w62]
        stop <- w64 stop-if-true
        w83 = TRUE  # append to file? (new file:F)
        w90 = i16 3 ("precision (6)")
        w113 = 0 ("index")
        # "WD"
        # "NA"
        # "N Photons"
        # "End Vector (mm)"
        # "End Position (mm)"
        # "Start Position (mm)"
        # "Distance (mm)"
        n19 = Build Path(base path=w138, name or relative path=w126) -> (appended path=w137:path)
        n20 = Compound Arithmetic op=MULTIPLY(w84, w85, w86) -> (w61:i32)
        n21 = call-poly <vilib>:"Read Delimited Spreadsheet.vi"("file path (dialog if empty)"=w137) -> ("all rows"=w125:string[][])  [unwired: 9 in, 5 out]
        n22 = feedback #1() -> (w87:dbl)
        n23 = Increment(x=w87) -> (x+1=w63:dbl)
        n24 = feedback-in #1(w63) -> ()
        n25 = Delete From Array(array=w125, length=9, index (row)=0) -> (deleted portion=w120:string[][], array with subset deleted=w115:string[][])  [unwired: 1 in]
        n26 = Fract/Exp String To Number(string=w115) -> (number=w122:dbl[][])  [unwired: 3 in, 1 out]
        n27 = Delete From Array(array=w120, index (row)=8) -> (deleted portion=w119:string[], array with subset deleted=w108:string[][])  [unwired: 2 in]
        n28 = Array Subset(array=w122, index (col)=6 ("index"), length (col)=3 ("length")) -> (w131:dbl[][])  [unwired: 2 in]
        n29 = Array Subset(array=w122, index (col)=9 ("index"), length (col)=3 ("length")) -> (w130:dbl[][])  [unwired: 2 in]
        n30 = Index Array(array=w122, index (col)=12 ("disabled index (col)")) -> (element=w116:dbl[])  [unwired: 1 in]
        n31 = Array Subset(array=w122, index (col)=0 ("index"), length (col)=3 ("length")) -> (w127:dbl[][])  [unwired: 2 in]
        n32 = Array Subset(array=w119, index=0, length=3) -> (w111:string[])
        n33 = Array Subset(array=w115, index (row)=w113, length (row)=1 ("length"), index (col)=w113, length (col)=3 ("length")) -> (w110:string[][])
        n34 = for {
          tunnel: w131 -> [w179] mode=indexing
          tunnel: w130 -> [w178] mode=indexing
          tunnel: w116 -> [w175] mode=indexing
          tunnel: [w173] -> w96 mode=indexing
          tunnel: w127 -> [w170] mode=indexing
          tunnel: w89 -> [w172]
          tunnel: w88 -> [w168]
          n35 = Array To Cluster "N=3"(array=w178) -> (cluster=w177:cluster{"[0]":dbl, "[1]":dbl, "[2]":dbl})
          n36 = Array To Cluster "N=3"(array=w179) -> (cluster=w176:cluster{"[0]":dbl, "[1]":dbl, "[2]":dbl})
          n37 = Array To Cluster "N=3"(array=w170) -> (cluster=w169:cluster{"[0]":dbl, "[1]":dbl, "[2]":dbl})
          n38 = call "ClassifyExitPhoton.vi"("WD (4)"=w168, "NA (1)"=w172, "V - Exit"=w177, "R - Exit"=w176, "R - Focal Point"=w169) -> ("Phi"=w174:dbl, "Photon State"=w171:T2)  [unwired: 5 in]
          n39 = Bundle("Photon State"=w171, "Phi"=w174, "String"=w175) -> (w173:T3)  [unwired: 1 in]
        }
        n40 = Build Array (concatenate)(w111, w110) -> (w109:string[][])
        n41 = Transpose 2D Array(2D array=w109) -> (transposed array=w107:string[][])
        n42 = Build Array (concatenate)(w108, w107) -> (w106:string[][])
        n43 = Transpose 2D Array(2D array=w106) -> (transposed array=w104:string[][])
        n44 = Sort 1D Array(array=w96) -> (sorted array=w98:T4)
        n45 = call "Utility - Delete Empty Rows or Columns.vi"("Delete Option"=T1."Delete Empty Rows", "Array In"=w104) -> ("Array Out"=w102:string[][])  [unwired: 1 in]
        "transposed array" <- w102
        n46 = for {
          N -> [w158]
          tunnel: w98 -> [w163] mode=indexing
          shift-right: [w160] -> w67
          shift-left: dbl[] [] -> [w159]
          tunnel: [w158] -> w76
          n47 = Unbundle(w163) -> ("Photon State"=w162:T2, "String"=w161:dbl)  [unwired: 1 out]
          n48 = case shown="\"Detected - Low Scattering\"" w162 {
            tunnel: w161 -> [w166 _]
            tunnel: [w165 w167] -> w160
            tunnel: w159 -> [w164 w167]
            frame "Detected - Low Scattering" {
              n49 = Build Array (concatenate)(w164, w166) -> (w165:dbl[])
            }
            frame Default {
            }
          }
        }
        n50 = Index Array(array=w102, index (row) #1=0 ("index (row)"), index (row) #2=1 ("index (row)")) -> (element #1=w71:string[], element #2=w95:string[])  [unwired: 2 in]
        n51 = Array Size(array=w96) -> (size(s)=w97:i32)
        n52 = for {
          tunnel: w103 -> [w157] mode=indexing
          tunnel: w67 -> [w153]
          tunnel: [w154] -> w99 mode=indexing
          tunnel: [w151] -> w79 mode=indexing
          tunnel: [w150] -> w78 mode=indexing
          n53 = Multiply(x=w153, y=w157) -> (x*y=w156:dbl[])
          n54 = Negate(x=w156) -> (-x=w155:dbl[])
          n55 = Power Of 10(x=w155) -> (10^x=w152:dbl[])
          n56 = Add Array Elements(numeric array=w152) -> (sum=w154:dbl)
          n57 = call <vilib>:"Std Deviation and Variance.vi"("X"=w152) -> ("mean"=w151:dbl, "standard deviation"=w150:dbl)  [unwired: 1 in, 1 out]
        }
        n58 = Number To Decimal String(number=w97) -> (decimal integer string=w94:string)  [unwired: 1 in]
        n59 = Number To Fractional String(number=w89, precision (6)=w90) -> (F-format string=w92:string)  [unwired: 2 in]
        n60 = Number To Fractional String(number=w88, precision (6)=w90) -> (F-format string=w91:string)  [unwired: 2 in]
        n61 = call <vilib>:"Std Deviation and Variance.vi"("X"=w67) -> ("mean"=w75:dbl, "standard deviation"=w74:dbl)  [unwired: 1 in, 1 out]
        n62 = Array Size(array=w67) -> (size(s)=w66:i32)
        n63 = call-poly "File Exists__ogtk.vi"("file path"=w70) -> ("exists"=w73:bool)  [unwired: 6 in, 1 out]
        n64 = case shown="False" w73 {
          tunnel: w72 -> [w144 _]
          tunnel: w71 -> [w143 _]
          tunnel: w70 -> [w142 w149]
          tunnel: [w141 w149] -> w69
          tunnel: [w140 errorcluster {"status"=FALSE, "code"=0, "source"=""} ("error out")] -> w68
          frame False {
            # "Header"
            n65 = Build Array (concatenate)(w143, "N Photons", "NA", "WD", w144) -> (w139:string[])
            "Header" <- w139
            n66 = call-poly <vilib>:"Write Delimited Spreadsheet.vi"("file path (dialog if empty)"=w142, "1D data"=w139) -> ("new file path (Not A Path if cancelled)"=w141:path, "error out"=w140:errorcluster)  [unwired: 12 in]
          }
          frame True {
          }
        }
        n67 = Divide(x=w99, y=w76) -> (x/y=w80:dbl[])
        n68 = Build Array (concatenate)(w66, w75, w74, w80, w79, w78) -> (w77:dbl[])
        n69 = Number To Fractional String(number=w77) -> (F-format string=w93:string[])  [unwired: 3 in]
        n70 = Build Array (concatenate)(w95, w94, w92, w91, w93) -> (w82:string[])
        n71 = call-poly <vilib>:"Write Delimited Spreadsheet.vi"("file path (dialog if empty)"=w69, "1D data"=w82, "append to file? (new file:F)"=w83, "error in (no error)"=w68) -> ("error out"=w64:errorcluster)  [unwired: 10 in, 1 out]
        n72 = call "Time to End.vi"("Trigger"=w64, "Start Time (ms)"=w62, "i"=w63, "N"=w61) -> ("Time to End"=→"Time to End":cluster{"Time To End":dbl, "unit":string}, "Percent Complete"=→"Percent Complete":dbl)  [unwired: 3 in, 3 out]
      }
    }
  }
  "error out" <- w3
